vi "Plugin.Get Timing.vi"(11 "Plugin in":refnum<class "Plugin.lvclass">) -> (2 "Timing":refnum<class "Timing.lvclass">, 3 "Plugin out":refnum<class "Plugin.lvclass">)   [LabVIEW 2017, in "DSF.Engine.lvlib" / "Plugin.lvclass"]
uses:
  Plugin.lvclass
  Timing/Timing.lvclass
  Plugin.lvclass/Plugin.ctl
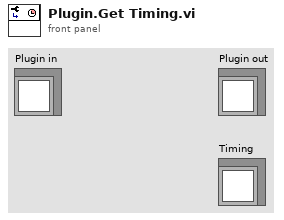
[diagram p1: front panel]
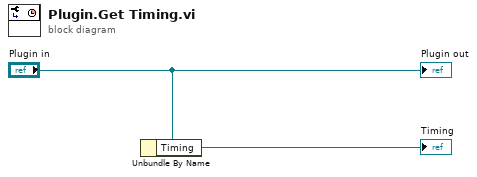
[diagram p0: block diagram]
diagram:
  n1 = Unbundle By Name("Plugin in") -> ("Timing"=→"Timing":refnum<class "Timing.lvclass">)
  "Plugin out" <- "Plugin in"
